vi "optionsAcq_spectrumType.vi"(8 "error in (no error)":errorcluster, 9 "readWrite":enum16{"read", "write"}(ring), 10 "spectrum channel type":T1, 11 "Thorlabs_OSA300_64 in":refnum<class "OSA300.lvclass">) -> (0 "error out":errorcluster, 2 "spectrum channel out":T1, 3 "Thorlabs_OSA300_64 out":refnum<class "OSA300.lvclass">)   [LabVIEW 2010, in "OSA300.lvclass"]
uses:
  OSA300.lvclass
  _misc/Thorlabs_FTS_misc.llb/channelType_spectrum.ctl
  OSA20X_misc.lvlib
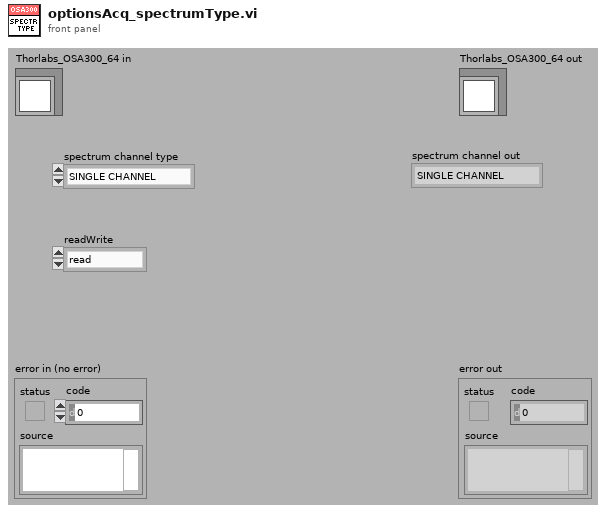
[diagram p1: front panel]
types:
  T1 = typedef "OSA20X_misc.lvlib/channelType_spectrum.ctl" = enum16{"SINGLE CHANNEL", "STICHED"}
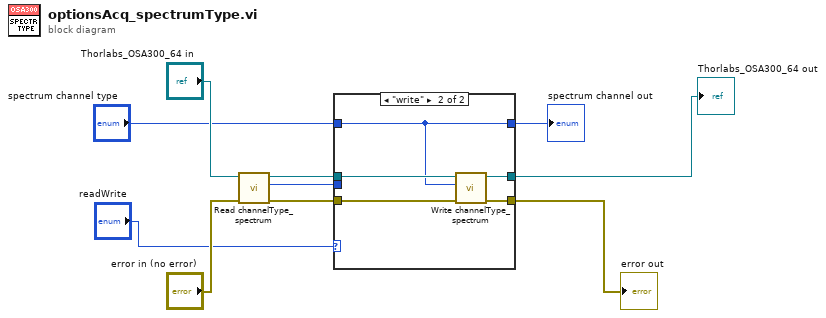
[diagram p0: block diagram]
diagram:
  n1 = call "Read channelType_spectrum.vi"("error in (no error)"="error in (no error)", "OSA300 in"="Thorlabs_OSA300_64 in") -> ("error out"=w8:errorcluster, "channelType_spectrum"=w7:T1, "OSA300 out"=w5:refnum<class "OSA300.lvclass">)  [unwired: 7 in]
  n2 = case shown="\"write\"" "readWrite" {
    tunnel: w5 -> [w13 w18]
    tunnel: "spectrum channel type" -> [_ w17]
    tunnel: [w11 w17] -> w3
    tunnel: w8 -> [w12 w16]
    tunnel: [w13 w15] -> w2
    tunnel: [w12 w14] -> w1
    tunnel: w7 -> [w11 _]
    frame "read", Default {
    }
    frame "write" {
      n3 = call "Write channelType_spectrum.vi"("error in (no error)"=w16, "channelType_spectrum"=w17, "OSA300 in"=w18) -> ("error out"=w14:errorcluster, "OSA300 out"=w15:refnum<class "OSA300.lvclass">)  [unwired: 7 in]
    }
  }
  "error out" <- w1
  "Thorlabs_OSA300_64 out" <- w2
  "spectrum channel out" <- w3
